vi "Controller Algorithm.vi"(8 "Heater Output":refnum<class "Abs_Boolean.lvclass">, 9 "Lower Limit":refnum<class "Abs_Double Float.lvclass">, 10 "Upper Limit":refnum<class "Abs_Double Float.lvclass">, 11 "Reading":refnum<class "Abs_Double Float.lvclass">) -> (3 "Node Out":refnum<class "bt_Node.lvclass">)   [LabVIEW 2021]
uses:
  Source/Support/Nodes/abs_Node/bt_Node.lvclass
  <vilib>/TSA/Abstract Data Classes/Abs_Types/Double Float/Abs_Double Float.lvclass
  C:/Program Files (x86)/National Instruments/LabVIEW 2021/vi.lib/TSA/Abstract Data Classes/Abs_Types/Numeric/Abs_Numeric.lvclass
  <vilib>/TSA/Abstract Data Classes/Abs_Types/Boolean/Abs_Boolean.lvclass
  C:/Program Files (x86)/National Instruments/LabVIEW 2021/vi.lib/TSA/Abstract Data Classes/Abs_Types/Type/Abs_Type.lvclass
  BT Abstract Type/abs_Type Leaf/abs_Type Leaf.lvclass/abs_Type Leaf.ctl
  BT Abstract Type/abs_Type Leaf/Properties/Write Value Class.vi
  BT Abstract Type/Test Boolean/Test Boolean.lvclass
  C:/Users/Tim/Documents/GitHub/LV_Behaviour_Tree/Source/Support/Nodes/abs_Node/bt_Node.lvclass
  C:/Users/Tim/Documents/GitHub/LV_Behaviour_Tree/BT Abstract Type/abs_Type Leaf/abs_Type Leaf.lvclass
  <vilib>/TSA/Abstract Data Classes/Functions/Compare/Support/Greater/DBL/Method.vi
  <vilib>/TSA/Abstract Data Classes/Functions/Compare/Support/Less/DBL/Method.vi
  BT Abstract Type/BT AbsType.lvlib
  Source/BT.lvlib
  <vilib>/TSA/Abstract Data Classes/Functions/Compare/Support/Less/DBL/Less_DBL.lvclass
  C:/Program Files (x86)/National Instruments/LabVIEW 2021/vi.lib/TSA/Abstract Data Classes/Abs_Types/Floating Point/Abs_Floating Point.lvclass
  C:/Program Files (x86)/National Instruments/LabVIEW 2021/vi.lib/TSA/Abstract Data Classes/Abs_Types/Value/Abs_Value.lvclass
  C:/Program Files (x86)/National Instruments/LabVIEW 2021/vi.lib/TSA/Abstract Data Classes/Abs_Types/Double Float/Abs_Double Float.lvclass
  <vilib>/TSA/Abstract Data Classes/Functions/Compare/Support/Greater/DBL/Greater_DBL.lvclass
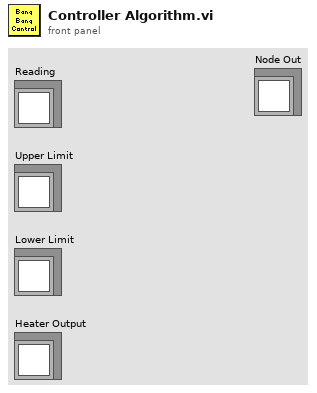
[diagram p1: front panel]
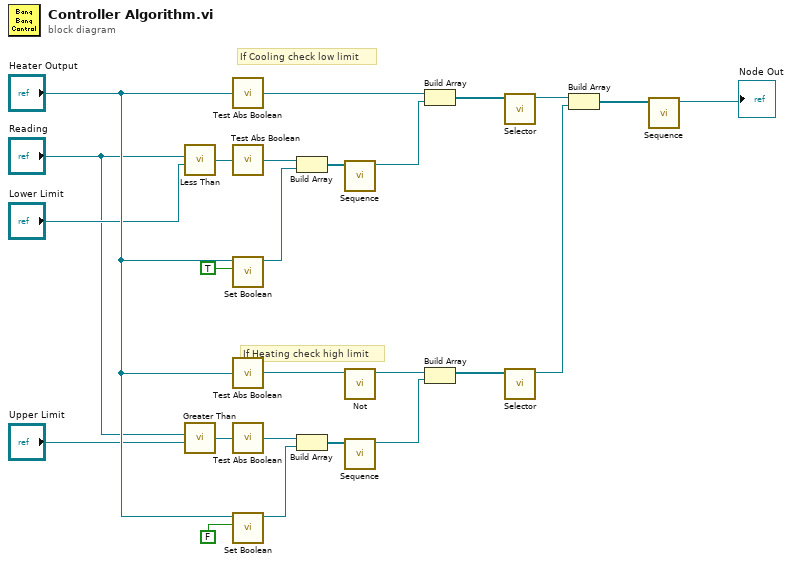
[diagram p0: block diagram]
diagram:
  # "If Heating check high limit"
  # "If Cooling check low limit"
  n1 = call-poly <vilib>:"Less Than.vi"("Value B"="Lower Limit", "Value A"="Reading") -> ("Result"=w6:refnum<class "Abs_Boolean.lvclass">)  [unwired: 4 in]
  n2 = call-poly <vilib>:"Greater Than.vi"("Value B"="Upper Limit", "Value A"="Reading") -> ("Result"=w2:refnum<class "Abs_Boolean.lvclass">)  [unwired: 4 in]
  n3 = call "Test Abs Boolean.vi"("Abs_Boolean.lvclass"="Heater Output") -> ("abs_Node"=w10:refnum<class "bt_Node.lvclass">)  [unwired: 4 in]
  n4 = call "Test Abs Boolean.vi"("Abs_Boolean.lvclass"=w6) -> ("abs_Node"=w7:refnum<class "bt_Node.lvclass">)  [unwired: 4 in]
  n5 = call "Set Boolean.vi"("Boolean Value"=TRUE, "Abs_Boolean.lvclass"="Heater Output") -> ("Node"=w21:refnum<class "bt_Node.lvclass">)  [unwired: 9 in]
  n6 = call "Test Abs Boolean.vi"("Abs_Boolean.lvclass"="Heater Output") -> ("abs_Node"=w9:refnum<class "bt_Node.lvclass">)  [unwired: 4 in]
  n7 = call "Test Abs Boolean.vi"("Abs_Boolean.lvclass"=w2) -> ("abs_Node"=w1:refnum<class "bt_Node.lvclass">)  [unwired: 4 in]
  n8 = call "Set Boolean.vi"("Boolean Value"=FALSE, "Abs_Boolean.lvclass"="Heater Output") -> ("Node"=w18:refnum<class "bt_Node.lvclass">)  [unwired: 9 in]
  n9 = Build Array(w7, w21) -> (w24:refnum<class "bt_Node.lvclass">[])
  n10 = Build Array(w1, w18) -> (w15:refnum<class "bt_Node.lvclass">[])
  n11 = call "Sequence.vi"("Nodes"=w24) -> ("Node"=w23:refnum<class "bt_Node.lvclass">)  [unwired: 10 in]
  n12 = call "Not.vi"("Node In"=w9) -> ("Node"=w8:refnum<class "bt_Node.lvclass">)  [unwired: 10 in]
  n13 = call "Sequence.vi"("Nodes"=w15) -> ("Node"=w16:refnum<class "bt_Node.lvclass">)  [unwired: 10 in]
  n14 = Build Array(w10, w23) -> (w25:refnum<class "bt_Node.lvclass">[])
  n15 = Build Array(w8, w16) -> (w12:refnum<class "bt_Node.lvclass">[])
  n16 = call "Selector.vi"("Nodes"=w25) -> ("Node"=w20:refnum<class "bt_Node.lvclass">)  [unwired: 10 in]
  n17 = call "Selector.vi"("Nodes"=w12) -> ("Node"=w11:refnum<class "bt_Node.lvclass">)  [unwired: 10 in]
  n18 = Build Array(w20, w11) -> (w19:refnum<class "bt_Node.lvclass">[])
  n19 = call "Sequence.vi"("Nodes"=w19) -> ("Node"=→"Node Out":refnum<class "bt_Node.lvclass">)  [unwired: 10 in]
